vi "rqcBob Test Launcher.vi"() -> ()   [LabVIEW 2018]
uses:
  rqcBob Classes/rqcBob/rqcBob.lvclass
panel:
  in  "Key Distribution":bool
  in  "Alice Modulator Level Test":bool
  in  "Alice Delay Line Test":bool
  in  "Mudulator Level Test":bool
  in  "Detector Window Test":bool
  in  "Channel Test":bool
  in  "Stop":bool
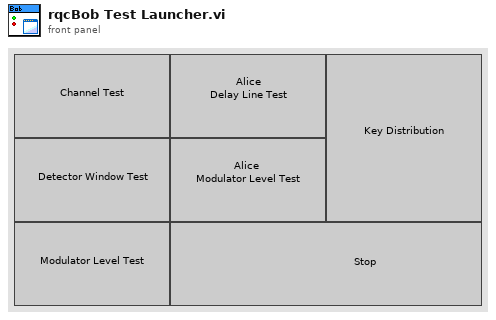
[diagram p1: front panel]
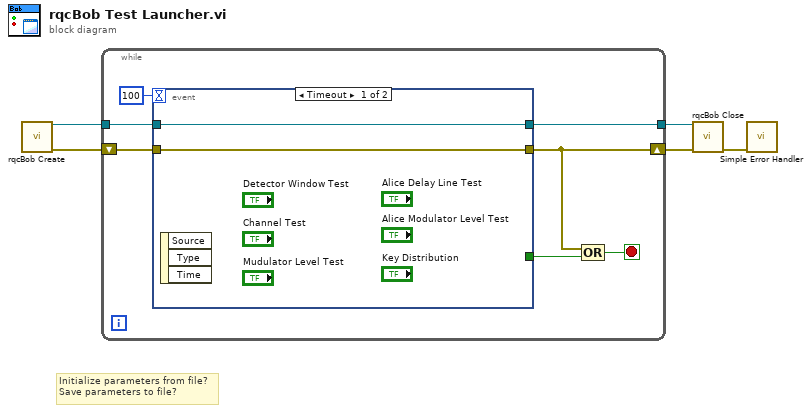
[diagram p0: block diagram]
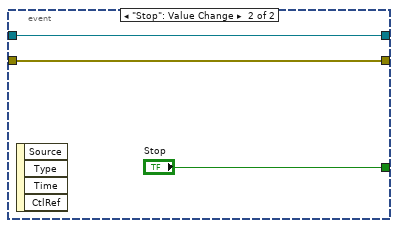
[diagram p2: hidden frame]
diagram:
  # "Initialize parameters from file?\nSave parameters to file?"
  n1 = call "rqcBob Create.vi"() -> ("rqcBob out"=w5:refnum<class "rqcBob.lvclass">, "error out"=w3:errorcluster)  [unwired: 14 in]
  n2 = while {
    tunnel: w5 -> [w12]
    tunnel: [w11] -> w4
    shift-right: [w6] -> w2
    shift-left: w3 -> [w10]
    stop <- w7 stop-if-true
    n3 = event shown="[0] Timeout" {
      selector: _ -> [_ _]
      dyn-events: _ -> [_ _]
      timeout: 100 -> [_ _]
      tunnel: [w14 w16] -> w11
      tunnel: w12 -> [w14 w16]
      tunnel: w10 -> [w13 w15]
      tunnel: [w13 w15] -> w6
      tunnel: [_ "Stop"] -> w9
      event Timeout {
        n4 = event-data() -> ()  [unwired: 1 in, 3 out]
      }
      event "Stop": Value Change {
        n5 = event-data() -> ()  [unwired: 1 in, 4 out]
      }
    }
    n6 = Compound Arithmetic op=OR(w6, w9) -> (w7:bool)
  }
  n7 = call-dynamic "rqcBob Close.vi"("rqcBob in"=w4, "error in"=w2) -> ("error out"=w1:errorcluster)  [unwired: 13 in]
  n8 = call <vilib>:"Simple Error Handler.vi"("error in (no error)"=w1) -> ()  [unwired: 4 in, 5 out]
